vi "Preference.vi"(7 "Auto Defrag":bool, 8 "error in":errorcluster, 9 "Buffer size":u32=1000 min=1 step=1 format="%d data", 10 "Sampling Period":u32=100 min=1 step=1 format="%.0f msec", 11 "Server Name":string="localhost") -> (0 "error out":errorcluster, 1 "Buffer size":i64, 2 "Sampling Period":i64, 3 "Server Name":string, 5 "Auto Defrag":bool)   [LabVIEW 2014]
doc: "<B>Copyrights</B>: (c) Ehsan Peymani 2015. All rights reserved.\n\nThis subVI updates the settings for data logging."
panel:
  in  "update":bool
  # "Logging Preference"
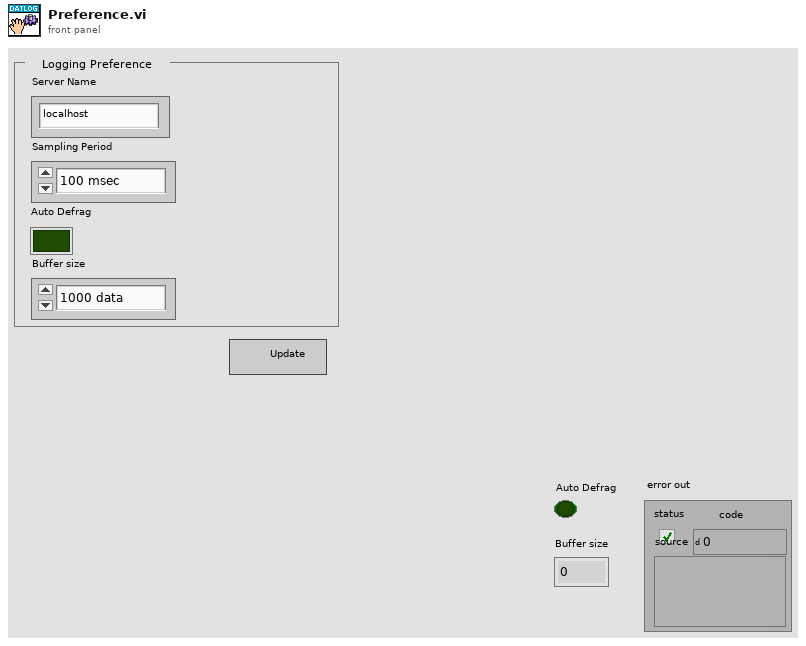
[diagram p1: front panel]
types:
  T1 = typedef "eventvkey.ctl" = enum16{"ASCII", "Enter", "Return", "Shift", "Ctrl", "Alt", "Cmd", "Opt", "Caps", "NumLock", "Clear", "Break", "Up", "Down", "Left", "Right", "Insert", "Delete", "Home", "End", "PageUp", "PageDown", "Escape", "Help", "Pause", "ScrollLock", "F1", "F2", "F3", "F4", "F5", "F6", "F7", "F8", "F9", "F10", "F11", "F12", "F13", "F14", "F15", "F16", "F17", "F18", "F19", "F20", "F21", "F22", "F23", "F24", "Play", "VolumeUp", "VolumeDown", "Mute", "Two Byte Char"}
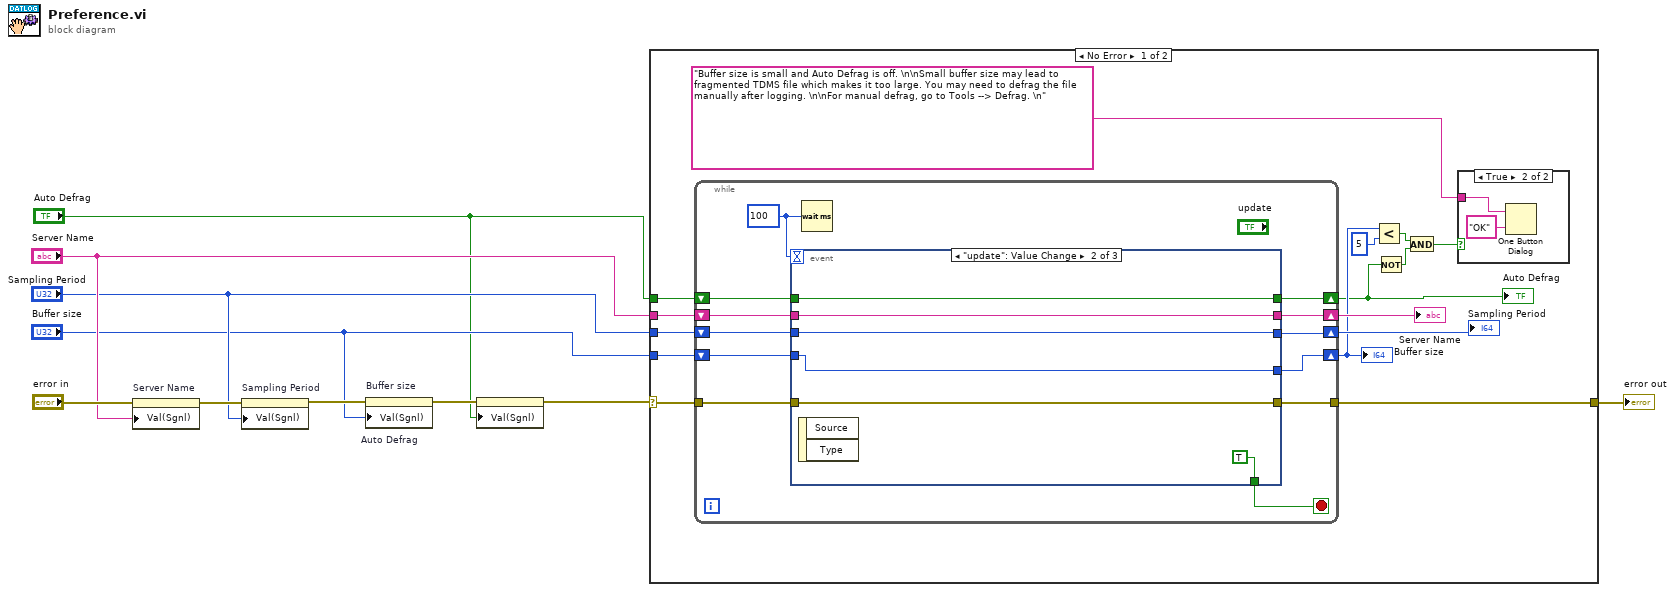
[diagram p0: block diagram]
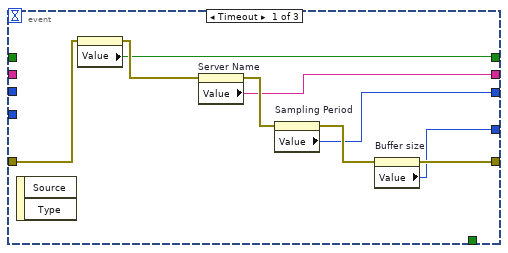
[diagram p3: hidden frame]
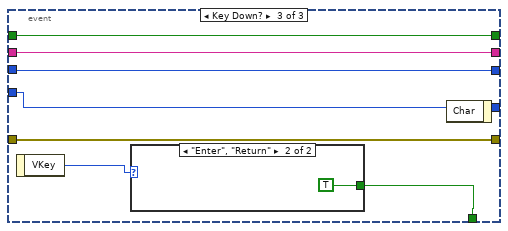
[diagram p4: hidden frame]
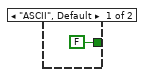
[diagram p5: hidden frame]
diagram:
  n1 = property on="Server Name" class="Str"(error in="error in", "Val(Sgnl)"="Server Name") -> (error out=w8:errorcluster)  [unwired: 1 in, 1 out]
  n2 = property on="Sampling Period" class="DigNum (strict)"(error in=w8, "Val(Sgnl)"="Sampling Period") -> (error out=w7:errorcluster)  [unwired: 1 in, 1 out]
  n3 = property on="Buffer size" class="DigNum (strict)"(error in=w7, "Val(Sgnl)"="Buffer size") -> (error out=w3:errorcluster)  [unwired: 1 in, 1 out]
  n4 = property on="Auto Defrag" class="Bool (strict)"(error in=w3, "Val(Sgnl)"="Auto Defrag") -> (error out=w2:errorcluster)  [unwired: 1 in, 1 out]
  n5 = case shown="No Error" w2 {
    selector: w2 -> [w25 w64]
    tunnel: [w24 w64] -> w10
    tunnel: "Server Name" -> [w23 _]
    tunnel: "Sampling Period" -> [w22 _]
    tunnel: "Buffer size" -> [w21 _]
    tunnel: "Auto Defrag" -> [w20 _]
    frame No Error {
      n6 = while {
        shift-right: [w36] -> w19
        shift-left: w23 -> [w39]
        shift-right: [w35] -> w17
        shift-left: w21 -> [w38]
        tunnel: w25 -> [w33]
        tunnel: [w32] -> w24
        shift-right: [w30] -> w18
        shift-left: w22 -> [w31]
        shift-right: [w28] -> w15
        shift-left: w20 -> [w29]
        stop <- w34 stop-if-true
        w37 = u32 100 ("milliseconds to wait")
        n7 = event shown="[1] \"update\": Value Change" {
          selector: _ -> [_ _ _]
          dyn-events: _ -> [_ _ _]
          timeout: w37 -> [_ _ _]
          tunnel: w39 -> [_ w53 w58]
          tunnel: w38 -> [_ w52 w60]
          tunnel: [w45 w53 w58] -> w36
          tunnel: [w43 w52 w60] -> w35
          tunnel: [_ TRUE w56] -> w34
          tunnel: w33 -> [w42 w51 w61]
          tunnel: [w46 w51 w61] -> w32
          tunnel: w31 -> [_ w50 w59]
          tunnel: [w44 w50 w59] -> w30
          tunnel: w29 -> [_ w49 w57]
          tunnel: [w40 w49 w57] -> w28
          event Timeout {
            n8 = event-data() -> ()  [unwired: 1 in, 2 out]
            n9 = property on="Auto Defrag" class="Bool (strict)"(error in=w42) -> (error out=w41:errorcluster, "Value"=w40:bool)  [unwired: 1 in, 1 out]
            n10 = property on="Server Name" class="Str"(error in=w41) -> (error out=w48:errorcluster, "Value"=w45:string)  [unwired: 1 in, 1 out]
            n11 = property on="Sampling Period" class="DigNum (strict)"(error in=w48) -> (error out=w47:errorcluster, "Value"=w44:u32)  [unwired: 1 in, 1 out]
            n12 = property on="Buffer size" class="DigNum (strict)"(error in=w47) -> (error out=w46:errorcluster, "Value"=w43:u32)  [unwired: 1 in, 1 out]
          }
          event "update": Value Change {
            n13 = event-data() -> ()  [unwired: 1 in, 2 out]
          }
          event Key Down? {
            n14 = event-data() -> ("VKey"=w55:T1)  [unwired: 1 in]
            n15 = case shown="\"Enter\", \"Return\"" w55 {
              tunnel: [FALSE TRUE] -> w56
              frame "ASCII", Default {
              }
              frame "Enter", "Return" {
              }
            }
            n16 = event-data() -> ()  [unwired: 2 in, 1 out]
          }
        }
        n17 = Wait (ms)(milliseconds to wait=w37) -> ()  [unwired: 1 out]
      }
      "Auto Defrag" <- w15
      "Server Name" <- w19
      "Sampling Period" <- w18
      "Buffer size" <- w17
      n18 = Less?(x=w17, y=i64 5) -> (x < y?=w14:bool)
      n19 = Not(x=w15) -> (.not. x?=w13:bool)
      n20 = And(x=w14, y=w13) -> (x .and. y?=w12:bool)
      n21 = case shown="True" w12 {
        tunnel: "Buffer size is small and Auto Defrag is off. \n\nSmall buffer size may lead to fragmented TDMS file which makes it too large. You may need to defrag the file manually after logging. \n\nFor manual defrag, go to Tools --> Defrag. \n" -> [_ w27]
        frame False {
        }
        frame True {
          n22 = One Button Dialog(message=w27, button name ("OK")="OK") -> ()  [unwired: 1 out]
        }
      }
    }
    frame Error {
    }
  }
  "error out" <- w10
